vi "On Data Message.vi"(8 "error in (no error)":errorcluster, 11 "This":refnum<class "WebSocket.lvclass">) -> (0 "error out":errorcluster, 3 "This out":refnum<class "WebSocket.lvclass">)   [LabVIEW 2017, in "WebSocket.lvclass"]
uses:
  WebSocket.lvclass
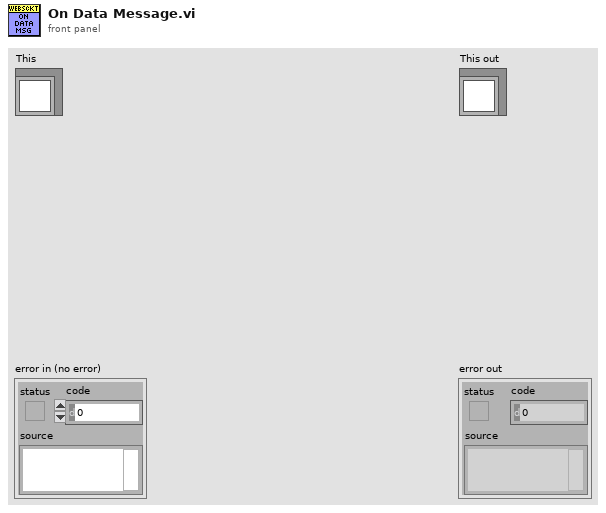
[diagram p1: front panel]
types:
  T1 = typedef "WebSocket.lvclass/ObjectAttributes.ctl" = cluster{"Socket":refnum<k5>, "Thread":refnum<vi>, "From Socket":refnum<queue>, "To Socket":refnum<queue>, "Rx Stats in Progress":variant, "Rx Stats":variant, "Tx Stats in Progress":variant, "Tx Stats":variant}
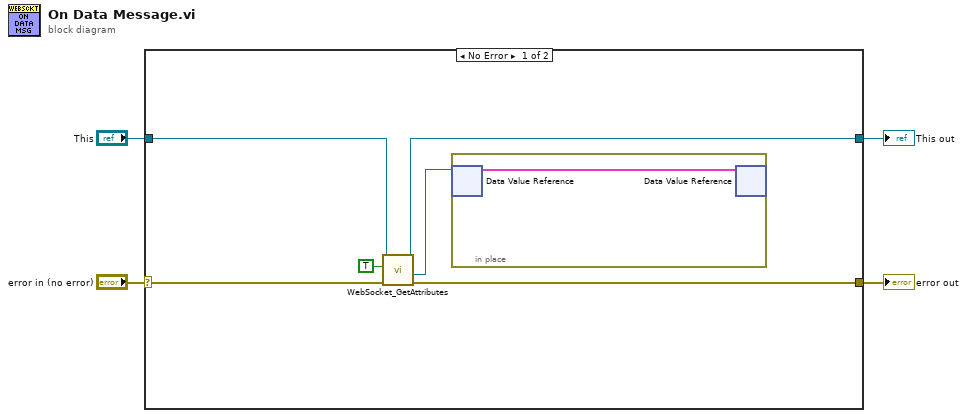
[diagram p0: block diagram]
diagram:
  n1 = case shown="No Error" "error in (no error)" {
    selector: "error in (no error)" -> [w5 w13]
    tunnel: [w9 w13] -> w3
    tunnel: [w8 w12] -> w1
    tunnel: "This" -> [w10 w12]
    frame No Error {
      n2 = call "WebSocket_GetAttributes.vi"("error in (no error)"=w5, "OnlyGetDvrReference(False)"=TRUE, "reference in"=w10) -> ("error out"=w9:errorcluster, "DataRef"=w6:refnum<data-value>, "reference out"=w8:refnum<class "WebSocket.lvclass">)  [unwired: 5 in, 1 out]
      n3 = in-place {
        n4 = in-place-dvr #1(w6) -> (w11:T1)  [unwired: 1 out]
        n5 = in-place-dvr #1(w11) -> ()  [unwired: 2 out]
      }
    }
    frame Error {
    }
  }
  "error out" <- w3
  "This out" <- w1
